vi "RotationScan.vi"(9 "Theta":dbl, 10 "w":dbl, 11 "h":dbl) -> (2 "w2":dbl, 3 "h2":dbl)   [LabVIEW 2016]
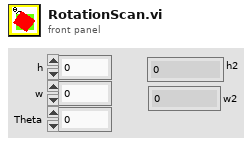
[diagram p1: front panel]
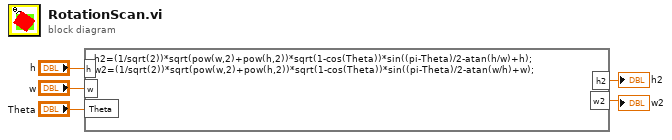
[diagram p0: block diagram]
diagram:
  n1 = formula code="h2=(1/sqrt(2))*sqrt(pow(w,2)+pow(h,2))*sqrt(1-cos(Theta))*sin((pi-Theta)/2-atan(h/w)+h);\nw2=(1/sqrt(2))*sqrt(pow(w,2)+pow(h,2))*sqrt(1-cos(Theta))*sin((pi-Theta)/2-atan(w/h)+w);"("h"="h", "w"="w", "Theta"="Theta") -> ("h2"=→"h2":dbl, "w2"=→"w2":dbl)
